vi "Day 3b.vi"() -> ()   [LabVIEW 2020]
uses:
  5c9fd22b-518c-4546-9cbe-2a54d6278cda.vi
  <vilib>/regexp/Match Regular Expression.xnode
panel:
  out "sum":i32
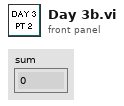
[diagram p1: front panel]
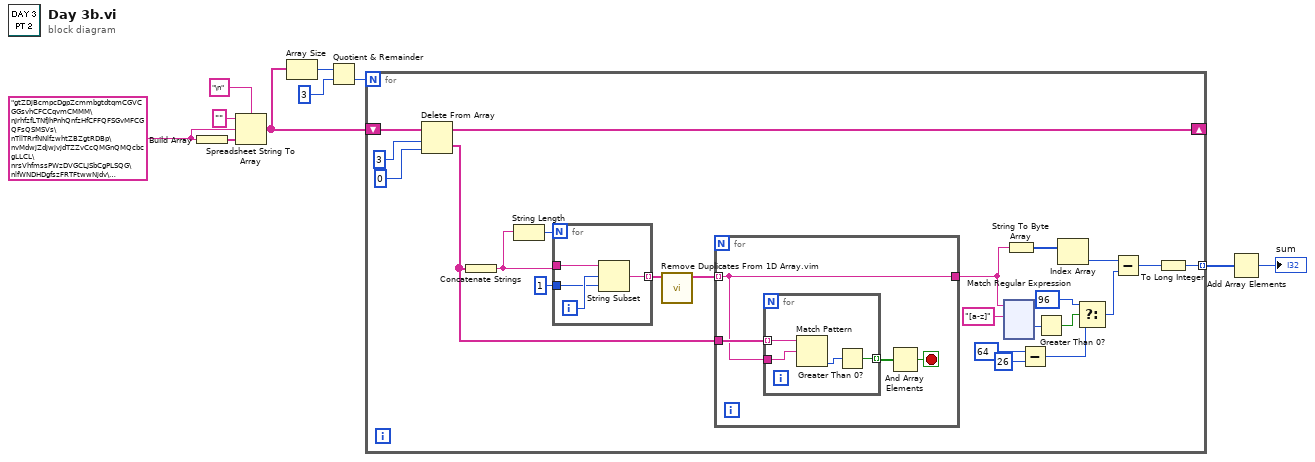
[diagram p0: block diagram]
diagram:
  w8 = "gtZDjBcmpcDgpZcmmbgtdtqmCGVCGGsvhCFCCqvmCMMM\nJrhfzfLTNfJhPnhQnfzHfCFFQFSGvMFCGQFsQSMSVs\nTllTRrfNNlfzwhtZBZgtRDBp\nvMdwjZdjwjvjdTZZvCcQMGnQMQcbcgLLCL\nrsVhfmssPWzDVGCLJSbCgPLSQG\nlfWNDHDgfszFRTFtwwNjdv\nGLPqVqdVGCLCdczjMjzMfzld\nJnWQvJDmvWBtlMzhrzfHQgcz\ntDtJDDDDtWRRmBwJwWtpPRsGCGScLPGSqspNCS\nChVzZzfNDzNJmBQfjjJfmH\nMrTMPMncGMJvPPvPWTbrMWvgmBgQwgdpwmdpdpjwpHQcdw\nSPvvvbqrFvMvZzJzsFVzVJNV\nmvBbvMFqbMMVVmtCBHpDdDPTDspdNWPDVP\nzjSfftcQtwtSfQSpNDppsNsjPNdRPP\nfgfStJShrgvvCLLv\nGmFnNNwbFFbhQQGQnGwwwfBgnMMqVDBZVVBMfMVzVz\nvWzRRHzTHcgfZDVfBgfH\nSSTvrvRcPpcvjFGwNGbNpbwQwz\nFFgbZZFZgFmpstLgmbtzqNrwVPlMPlSWWrMPNp\nQQhTv..."
  n1 = Build Array(w8) -> (w7:string[])
  n2 = Spreadsheet String To Array(delimiter (Tab)="\n", format string="", spreadsheet string=w8, array type (2D Dbl)=w7) -> (array=w3:string[])
  n3 = Array Size(array=w3) -> (size(s)=w6:i32)
  n4 = Quotient & Remainder(x=w6, y=3) -> (floor(x/y)=w5:i32)  [unwired: 1 out]
  n5 = for {
    N: w5 -> [_]
    shift-right: [w31] -> _
    shift-left: w3 -> [w30]
    tunnel: [w12] -> w1 mode=indexing
    n6 = Delete From Array(array=w30, length=3, index=0) -> (deleted portion=w25:string[], array with subset deleted=w31:string[])
    n7 = Concatenate Strings(w25) -> (w28:string)
    n8 = String Length(string=w28) -> (length=w29:i32)
    n9 = for {
      N: w29 -> [_]
      tunnel: w28 -> [w159]
      tunnel: [w157] -> w27 mode=indexing
      tunnel: 1 ("length (rest)") -> [w156]
      i -> [w158]
      n10 = String Subset(string=w159, offset (0)=w158, length (rest)=w156) -> (substring=w157:string)
    }
    n11 = call "Remove Duplicates From 1D Array.vim"("array"=w27) -> ("array with duplicates removed"=w26:string[])  [unwired: 10 in]
    n12 = for {
      tunnel: w26 -> [w149] mode=indexing
      tunnel: w25 -> [w151]
      tunnel: [w149] -> w17
      stop <- w148 stop-if-true
      n13 = for {
        tunnel: w151 -> [w155] mode=indexing
        tunnel: w149 -> [w154]
        tunnel: [w152] -> w150 mode=indexing
        n14 = Match Pattern(string=w155, regular expression=w154) -> (offset past match=w153:i32)  [unwired: 1 in, 3 out]
        n15 = Greater Than 0?(x=w153) -> (x > 0?=w152:bool)
      }
      n16 = And Array Elements(Boolean array=w150) -> (logical AND=w148:bool)
    }
    n17 = xnode "Match Regular Expression"("input string"=w17, "regular expression"="[a-z]") -> ("offset past match"=w23:i32)  [unwired: 4 in, 4 out]
    n18 = String To Byte Array(string=w17) -> (unsigned byte array=w16:u8[])
    n19 = Subtract(x=u8 64, y=u8 26) -> (x-y=w19:u8)
    n20 = Greater Than 0?(x=w23) -> (x > 0?=w21:bool)
    n21 = Index Array(array=w16) -> (element=w15:u8)  [unwired: 1 in]
    n22 = Select(t=u8 96, s=w21, f=w19) -> (s? t:f=w14:u8)
    n23 = Subtract(x=w15, y=w14) -> (x-y=w13:u8)
    n24 = To Long Integer(number=w13) -> (32bit integer=w12:i32)
  }
  n25 = Add Array Elements(numeric array=w1) -> (sum=→"sum":i32)
